vi "Set Visible Tab.vi"(8 "error in (no error)":errorcluster, 10 "Value":T1, 11 "UI in":refnum<class "UI.lvclass">) -> (0 "error out":errorcluster)   [LabVIEW 2020, in "AR Example.lvlib" / "UI.lvclass"]
uses:
  UI.lvclass
  Tab Control.ctl
  UI.lvclass/UI.ctl
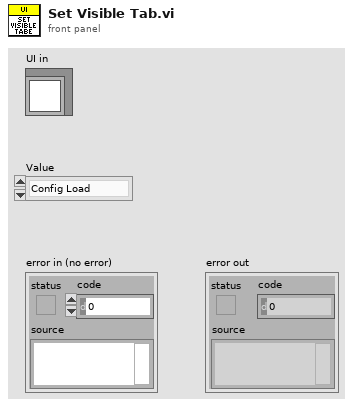
[diagram p1: front panel]
types:
  T1 = typedef "AR Example.lvlib/UI.lvclass/Tab Control.ctl" = enum8{"Config Load", "Camera Selection", "Camera Calibration"}
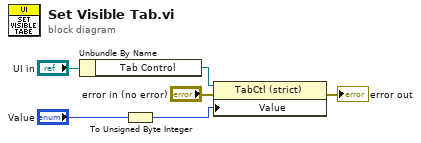
[diagram p0: block diagram]
diagram:
  n1 = Unbundle By Name("UI in") -> ("Tab Control"=w5:refnum<vi>)
  n2 = To Unsigned Byte Integer(number="Value") -> (unsigned 8bit integer=w2:u8)
  n3 = property class="TabCtl (strict)"(reference=w5, error in="error in (no error)", "Value"=w2) -> (error out=→"error out":errorcluster)  [unwired: 1 out]
